vi "hv_relay.vi"(8 "error in":errorcluster, 9 "data":bool, 11 "Micron config":T1) -> (0 "error out":errorcluster)   [LabVIEW 2010]
uses:
  initialization/micron_config.ctl
  <vilib>/DAQmx/write.llb/DAQmx Write (Digital Bool 1Line 1Point).vi
  asap/labview/initialization/globals.vi
  <vilib>/daqmx/miscellaneous.llb/DAQmx Fill In Error Info.vi
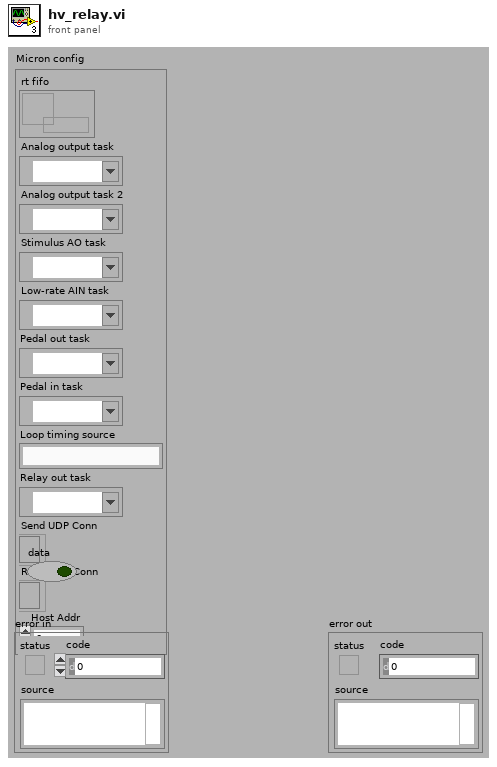
[diagram p1: front panel]
types:
  T1 = typedef "micron_config.ctl" = cluster{"rt fifo":refnum<k33>, "Analog output task":refnum<k21>, "Analog output task 2":refnum<k21>, "Stimulus AO task":refnum<k21>, "Low-rate AIN task":refnum<k21>, "Pedal out task":refnum<k21>, "Pedal in task":refnum<k21>, "Loop timing source":string, "Relay out task":refnum<k21>, "Send UDP Conn":refnum<k16>, "Recv UDP Conn":refnum<k16>, "Host Addr":dbl}
  T2 = enum16{"ASAP/Trigger", "ASAP/Finder", "ASAP/Micron", "ASAP/Micron 2"}
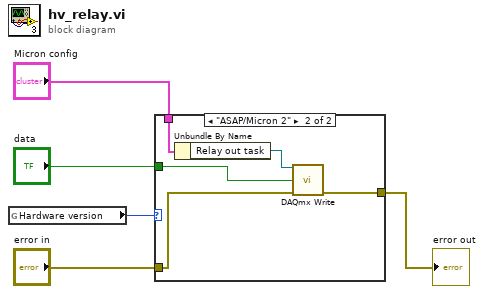
[diagram p0: block diagram]
diagram:
  n1 = global read "globals.vi" "Hardware version"() -> (w3:T2)
  n2 = case shown="\"ASAP/Micron 2\"" w3 {
    tunnel: "data" -> [_ w10]
    tunnel: "Micron config" -> [_ w9]
    tunnel: "error in" -> [w6 w8]
    tunnel: [w6 w7] -> w1
    frame "ASAP/Trigger", Default {
    }
    frame "ASAP/Micron 2" {
      n3 = Unbundle By Name(w9) -> ("Relay out task"=w11:refnum<k21>)
      n4 = call-poly <vilib>:"DAQmx Write.vi"("task/channels in"=w11, "data"=w10, "error in"=w8) -> ("error out"=w7:errorcluster)  [unwired: 1 in, 11 out]
    }
  }
  "error out" <- w1
